vi "MGI Handle PID (1 Chan).vi"(5 "dt (s)":dbl=-1.0 format="%.3f", 6 "PID State In":T1, 7 "output range":cluster{"output high":dbl, "output low":dbl}={"output high"=100.0, "output low"=-100.0} {"output low" format="%.2f"; "output high" format="%.2f"}, 9 "PID gains":T2={"proportional gain (Kc)"=1.0, "integral time (Ti, min)"=0.01, "derivative time (Td, min)"=0.0} {"derivative time (Td, min)" format="%.3f"; "integral time (Ti, min)" format="%.3f"; "proportional gain (Kc)" format="%.3f"}, 10 "process variable":dbl format="%.2f", 11 "setpoint":dbl format="%.2f") -> (2 "output":dbl format="%.2f", 3 "dt (s) out":dbl, 4 "PID State Out":T1)   [LabVIEW 2020]
doc: "This VI was coppied from National Instrument's PID.vi The National Instrument's PID.vi is a functional global that maintains PID state on uninitialized shift registers. This VI expects the PID state to be maintained by the caller. This approach is useful when each PID channel is handled in a loop. \n\nsupport@mooregoodideas.com\nwww.mooregoodideas.com"
uses:
  <userlib>/_MGI/Numeric/MGI Handle PID State Cluster.ctl
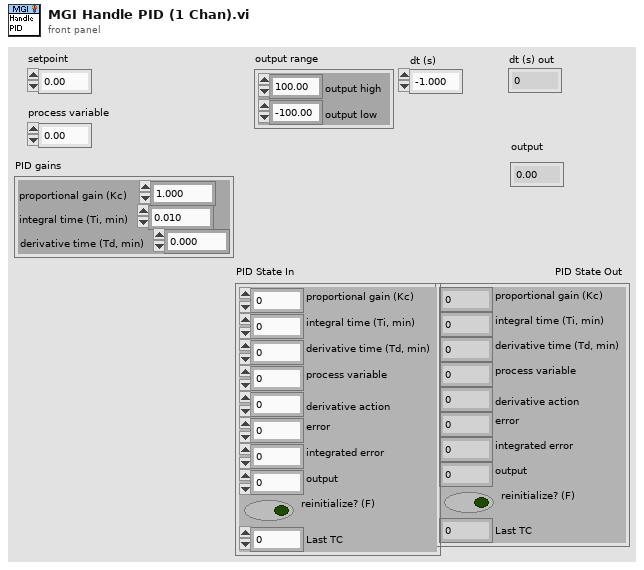
[diagram p1: front panel]
types:
  T1 = typedef "MGI Handle PID State Cluster.ctl" = cluster{"proportional gain (Kc)":dbl, "integral time (Ti, min)":dbl, "derivative time (Td, min)":dbl, "process variable":dbl, "derivative action":dbl, "error":dbl, "integrated error":dbl, "output":dbl, "reinitialize? (F)":bool, "Last TC":u32}
  T2 = cluster{"proportional gain (Kc)":dbl, "integral time (Ti, min)":dbl, "derivative time (Td, min)":dbl}
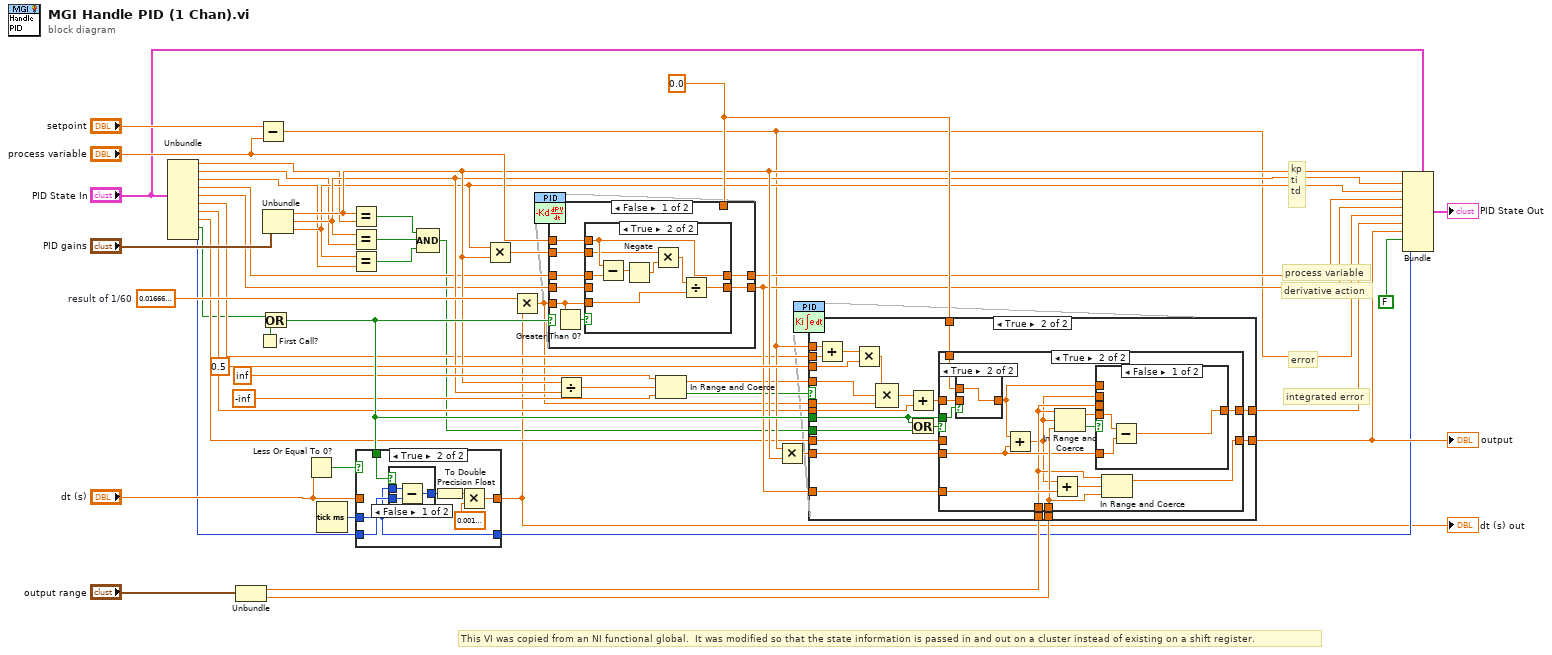
[diagram p0: block diagram]
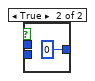
[diagram p3: hidden frame]
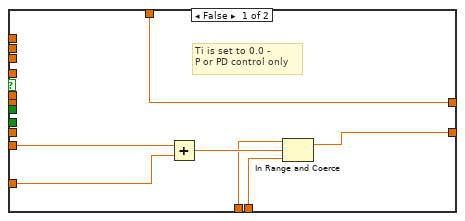
[diagram p4: hidden frame]
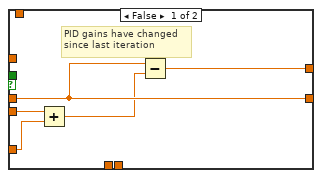
[diagram p5: hidden frame]
diagram:
  w37 = 0.0
  w46 = 0.016666666666666666  # result of 1/60
  # "This VI was copied from an NI functional global.  It was modified so that the state information is passed in and out on a cluster instead of existing on a shift register."
  # "derivative action"
  # "process variable"
  # "kp\nti\ntd"
  # "error"
  # "integrated error"
  n1 = Unbundle("PID State In") -> ("proportional gain (Kc)"=w27:dbl, "integral time (Ti, min)"=w26:dbl, "derivative time (Td, min)"=w25:dbl, "process variable"=w24:dbl, "derivative action"=w23:dbl, "error"=w21:dbl, "integrated error"=w20:dbl, "output"=w19:dbl, "reinitialize? (F)"=w18:bool, "Last TC"=w15:u32)
  n2 = Unbundle("output range") -> ("output high"=w48:dbl, "output low"=w47:dbl)
  n3 = First Call?() -> (First Call?: T/F=w36:bool)
  n4 = Subtract(x="setpoint", y="process variable") -> (x-y=w30:dbl)
  n5 = Or(x=w18, y=w36) -> (x .or. y?=w49:bool)
  n6 = Unbundle("PID gains") -> ("proportional gain (Kc)"=w35:dbl, "integral time (Ti, min)"=w34:dbl, "derivative time (Td, min)"=w33:dbl)
  n7 = Less Or Equal To 0?(x="dt (s)") -> (x <= 0?=w2:bool)
  n8 = Tick Count (ms)() -> (millisecond timer value=w1:u32)
  n9 = Equal?(x=w35, y=w27) -> (x = y?=w10:bool)
  n10 = Equal?(x=w34, y=w26) -> (x = y?=w9:bool)
  n11 = Equal?(x=w33, y=w25) -> (x = y?=w11:bool)
  n12 = case shown="True" w2 {
    tunnel: [w51 w55] -> w13
    tunnel: w15 -> [_ w54]
    tunnel: [w50 w52] -> w14
    tunnel: "dt (s)" -> [w51 _]
    tunnel: w49 -> [_ w53]
    tunnel: w1 -> [w50 w52]
    frame False {
    }
    frame True {
      n13 = case shown="False" w53 {
        tunnel: [w61 u32 0] -> w57
        tunnel: w54 -> [w60 _]
        tunnel: w52 -> [w59 _]
        frame False {
          n14 = Subtract(x=w59, y=w60) -> (x-y=w61:u32)
        }
        frame True {
        }
      }
      n15 = To Double Precision Float(number=w57) -> (double precision float=w56:dbl)
      n16 = Multiply(x=w56, y=0.0010000000474974513) -> (x*y=w55:dbl)
    }
  }
  "dt (s) out" <- w13
  n17 = Compound Arithmetic op=AND(w10, w9, w11) -> (w3:bool)
  n18 = Multiply(x=w33, y=w35) -> (x*y=w6:dbl)
  n19 = Multiply(x=w46, y=w13) -> (x*y=w12:dbl)
  n20 = case shown="False" w49 {
    tunnel: w24 -> [w70 _]
    tunnel: w6 -> [w67 _]
    tunnel: "process variable" -> [w69 w82]
    tunnel: [w66 w82] -> w32
    tunnel: [w68 w81] -> w31
    tunnel: w23 -> [w64 _]
    tunnel: w12 -> [w63 _]
    tunnel: w37 -> [_ w81]
    frame False {
      n21 = Greater Than 0?(x=w63) -> (x > 0?=w65:bool)
      n22 = case shown="True" w65 {
        tunnel: w70 -> [w72 w78]
        tunnel: w63 -> [_ w77]
        tunnel: w69 -> [_ w75]
        tunnel: [w71 w76] -> w68
        tunnel: w67 -> [_ w73]
        tunnel: [w72 w75] -> w66
        tunnel: w64 -> [w71 _]
        frame False {
          # "dt = 0 min"
        }
        frame True {
          n23 = Subtract(x=w75, y=w78) -> (x-y=w80:dbl)
          n24 = Negate(x=w80) -> (-x=w74:dbl)
          n25 = Multiply(x=w73, y=w74) -> (x*y=w79:dbl)
          n26 = Divide(x=w79, y=w77) -> (x/y=w76:dbl)
        }
      }
    }
    frame True {
    }
  }
  n27 = Divide(x=w35, y=w34) -> (x/y=w5:dbl)
  n28 = In Range and Coerce(upper limit=inf, x=w5, lower limit=-inf) -> (coerced(x)=w8:dbl, In Range?=w7:bool)
  n29 = Multiply(x=w30, y=w35) -> (x*y=w4:dbl)
  n30 = case shown="True" w7 {
    tunnel: w30 -> [_ w109]
    tunnel: w21 -> [_ w110]
    tunnel: w20 -> [_ w105]
    tunnel: [w83 w100] -> w29
    tunnel: w8 -> [_ w98]
    tunnel: w4 -> [w88 w103]
    tunnel: [w89 w99] -> w22
    tunnel: w19 -> [_ w101]
    tunnel: w31 -> [w87 w97]
    tunnel: w49 -> [_ w96]
    tunnel: w3 -> [_ w95]
    tunnel: w12 -> [_ w94]
    tunnel: w48 -> [w85 w92]
    tunnel: w47 -> [w84 w93]
    tunnel: 0.5 ("y") -> [_ w91]
    tunnel: w37 -> [w83 w90]
    frame False {
      # "Ti is set to 0.0 -\nP or PD control only"
      n31 = Add(x=w88, y=w87) -> (x+y=w86:dbl)
      n32 = In Range and Coerce(upper limit=w85, x=w86, lower limit=w84) -> (coerced(x)=w89:dbl)  [unwired: 1 out]
    }
    frame True {
      n33 = Add(x=w109, y=w110) -> (x+y=w108:dbl)
      n34 = Multiply(x=w108, y=w91) -> (x*y=w107:dbl)
      n35 = Compound Arithmetic op=MULTIPLY(w107, w98, w94) -> (w106:dbl)
      n36 = Add(x=w106, y=w105) -> (x+y=w104:dbl)
      n37 = Or(x=w96, y=w95) -> (x .or. y?=w102:bool)
      n38 = case shown="True" w102 {
        tunnel: w104 -> [_ w123]
        tunnel: w103 -> [w113 w118]
        tunnel: w101 -> [w115 _]
        tunnel: w96 -> [_ w125]
        tunnel: [w114 w120] -> w100
        tunnel: [w115 w128] -> w99
        tunnel: w97 -> [w112 w127]
        tunnel: w93 -> [_ w126]
        tunnel: w92 -> [_ w117]
        tunnel: w90 -> [_ w124]
        frame False {
          # "PID gains have changed\nsince last iteration"
          n39 = Add(x=w113, y=w112) -> (x+y=w111:dbl)
          n40 = Subtract(x=w115, y=w111) -> (x-y=w114:dbl)
        }
        frame True {
          n41 = case shown="True" w125 {
            tunnel: w124 -> [_ w135]
            tunnel: [w134 w135] -> w122
            tunnel: w123 -> [w134 _]
            frame False {
            }
            frame True {
            }
          }
          n42 = Add(x=w122, y=w118) -> (x+y=w116:dbl)
          n43 = Add(x=w116, y=w127) -> (x+y=w129:dbl)
          n44 = In Range and Coerce(upper limit=w117, x=w116, lower limit=w126) -> (coerced(x)=w119:dbl, In Range?=w121:bool)
          n45 = case shown="False" w121 {
            tunnel: w122 -> [_ w133]
            tunnel: [w130 w133] -> w120
            tunnel: w119 -> [w132 _]
            tunnel: w118 -> [w131 _]
            tunnel: w117 -> [_ _]
            tunnel: w116 -> [_ _]
            frame False {
              n46 = Subtract(x=w132, y=w131) -> (x-y=w130:dbl)
            }
            frame True {
            }
          }
          n47 = In Range and Coerce(upper limit=w117, x=w129, lower limit=w126) -> (coerced(x)=w128:dbl)  [unwired: 1 out]
        }
      }
    }
  }
  "output" <- w22
  n48 = Bundle(cluster="PID State In", "proportional gain (Kc)"=w35, "integral time (Ti, min)"=w34, "derivative time (Td, min)"=w33, "process variable"=w32, "derivative action"=w31, "error"=w30, "integrated error"=w29, "output"=w22, "reinitialize? (F)"=FALSE, "Last TC"=w14) -> (→"PID State Out":T1)
